vi "Send  Sensor Calibration.vi"(6 "Initialize/Close?":bool, 8 "Error In (No Error)":errorcluster, 9 "Sensor On/Off":bool, 10 "Sensor Address In":string="0", 11 "RS232 Port In":refnum<visa-resource-name>="COM11") -> (0 "Error Out":errorcluster, 1 "Sensor On/Off Response":bool, 2 "Address Out":string, 3 "RS232 Port Out":refnum<visa-resource-name>)   [LabVIEW 2016]
doc: "Sends an SDI-12 Send Identification Command, and returns the various attributes from the sensor's response.\n\nThe total size by the sensor must be 22-35 in size (inclusive), or this VI will return an error."
uses:
  SDI-12/SDI-12.lvlib
panel:
  out "Numeric":i32
  out "read buffer":string
  out "length":i32
  out "output 1":i16
  out "Command":string
  # "(c) 2008 National Instruments.  ALL RIGHTS RESERVED."
  # "The following are required,\nor are optional, for the sensors\nto respond with:"
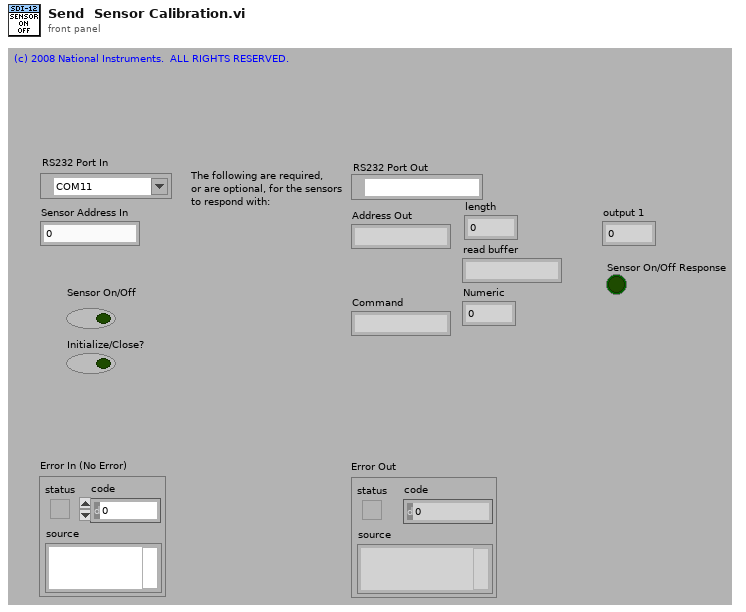
[diagram p1: front panel]
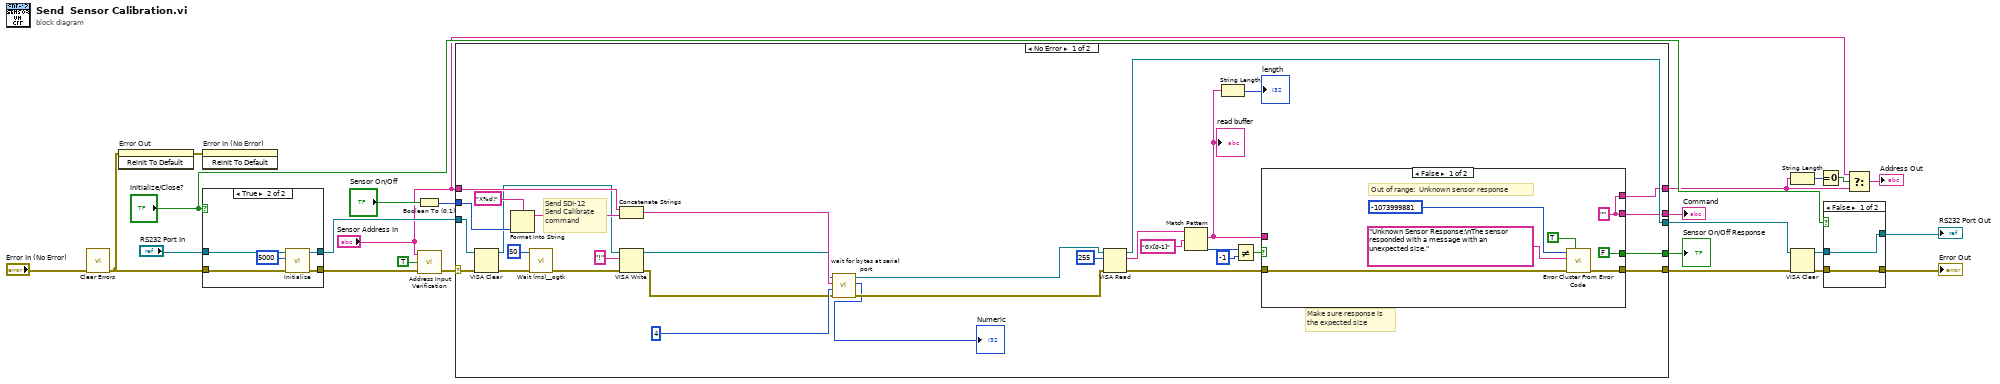
[diagram p0: block diagram]
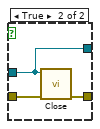
[diagram p2: hidden frame]
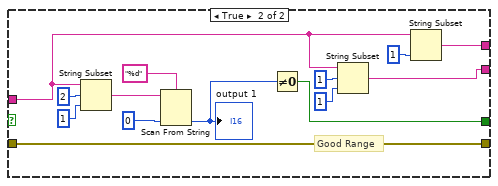
[diagram p4: hidden frame]
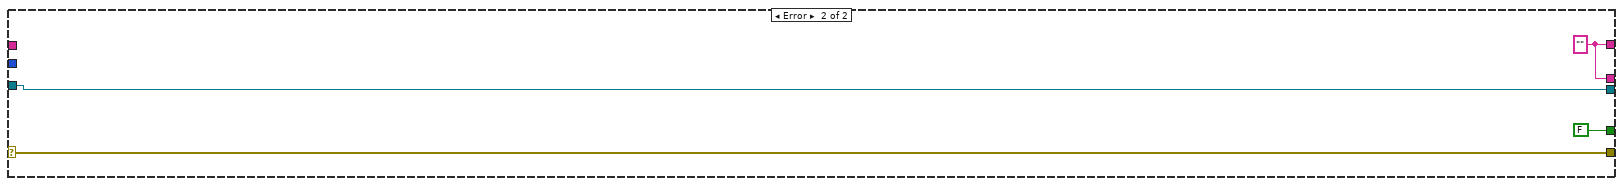
[diagram p5: hidden frame]
diagram:
  n1 = call <vilib>:"Clear Errors.vi"("error in (no error)"="Error In (No Error)") -> ("error out"=w5:errorcluster)  [unwired: 5 in, 1 out]
  n2 = invoke on="Error Out" class="Clust (strict)" method="Reinit To Default"(error in=w5) -> (error out=w4:errorcluster)  [unwired: 2 in, 2 out]
  n3 = invoke on="Error In (No Error)" class="Clust (strict)" method="Reinit To Default"(error in=w4) -> ()  [unwired: 2 in, 3 out]
  n4 = case shown="True" "Initialize/Close?" {
    tunnel: w5 -> [w26 w31]
    tunnel: [w26 w30] -> w16
    tunnel: "RS232 Port In" -> [w25 w29]
    tunnel: [w25 w28] -> w15
    frame False {
    }
    frame True {
      n5 = call "Initialize.vi"("Error In (No Error)"=w31, "General Settings:Timeout Value"=u32 5000, "RS232 Port In"=w29) -> ("Error Out"=w30:errorcluster, "RS232 Port Out"=w28:refnum<visa-resource-name>)  [unwired: 7 in]
    }
  }
  n6 = Boolean To (0,1)(Boolean="Sensor On/Off") -> (0, 1=w20:i16)
  n7 = call "Address Input Verification.vi"("Error In (No Error)"=w16, "Error if Bad? (True)"=TRUE ("error if bad? (True)"), "Sensor Address In (a)"="Sensor Address In") -> ("Error Out"=w24:errorcluster)  [unwired: 1 in, 1 out]
  n8 = case shown="No Error" w24 {
    selector: w24 -> [w50 w88]
    tunnel: [w58 w88] -> w2
    tunnel: "Sensor Address In" -> [w62 _]
    tunnel: w15 -> [w51 w87]
    tunnel: [w61 w87] -> w13
    tunnel: [w57 w86] -> w22
    tunnel: [w56 w86] -> w8
    tunnel: w20 -> [w55 _]
    tunnel: [w52 FALSE] -> w19
    frame No Error {
      # "Make sure response is\nthe expected size"
      # "Send SDI-12 \nSend Calibrate \ncommand"
      n9 = VISA Clear(VISA resource name=w51, error in (no error)=w50) -> (VISA resource name out=w41:refnum<visa-resource-name>, error out=w45:errorcluster)
      n10 = Format Into String(format string="X%d!", w55) -> (resulting string=w53:string)  [unwired: 2 in, 1 out]
      n11 = call "Wait (ms)__ogtk.vi"("error in (no error)"=w45, "milliseconds to wait"=u32 50) -> ("error out"=w42:errorcluster)  [unwired: 8 in, 1 out]
      n12 = Concatenate Strings(w62, w53) -> (w49:string)
      n13 = VISA Write(VISA resource name=w41, write buffer="!", error in (no error)=w42) -> (VISA resource name out=w33:refnum<visa-resource-name>, error out=w40:errorcluster)  [unwired: 1 out]
      n14 = call "wait for bytes at serial port.vi"("error in (no error)"=w40, "lower limit"=4, "String"=w49, "VISA Refnum in"=w33) -> ("error out"=w47:errorcluster, "loop"=→"Numeric":i32, "VISA Refnum out"=w48:refnum<visa-resource-name>)  [unwired: 4 in, 1 out]
      n15 = VISA Read(VISA resource name=w48, byte count=u32 255, error in (no error)=w47) -> (VISA resource name out=w61:refnum<visa-resource-name>, read buffer=w59:string, error out=w60:errorcluster)  [unwired: 1 out]
      n16 = Match Pattern(string=w59, regular expression="0X[0-1]") -> (match substring=w38:string, offset past match=w36:i32)  [unwired: 1 in, 2 out]
      "read buffer" <- w38
      n17 = String Length(string=w38) -> (length=→"length":i32)
      n18 = Not Equal?(x=w36, y=-1) -> (x != y?=w34:bool)
      n19 = case shown="False" w34 {
        tunnel: w60 -> [w66 w78]
        tunnel: [w67 w78] -> w58
        tunnel: w38 -> [_ w81]
        tunnel: [w65 w76] -> w57
        tunnel: [w65 w75] -> w56
        tunnel: [FALSE w71] -> w52
        frame False {
          w65 = "" ("read buffer")
          # "Out of range:  Unknown sensor response"
          n20 = call <vilib>:"Error Cluster From Error Code.vi"("show call chain? (False)"=TRUE, "error in (no error)"=w66, "error message (\"\")"="Unknown Sensor Response:\nThe sensor responded with a message with an unexpected size." ("error message (\"\")"), "error code (0)"=-1073999881) -> ("error out"=w67:errorcluster)  [unwired: 5 in]
        }
        frame True {
          # "Good Range"
          n21 = String Subset(string=w81, offset (0)=2, length (rest)=1 ("length (rest)")) -> (substring=w77:string)
          n22 = Scan From String(format string="%d", input string=w77, default 1=i16 0 ("default value 1")) -> (output 1=w72:i16)  [unwired: 2 in, 3 out]
          "output 1" <- w72
          n23 = Not Equal To 0?(x=w72) -> (x != 0?=w71:bool)
          n24 = String Subset(string=w81, offset (0)=1, length (rest)=1 ("length (rest)")) -> (substring=w76:string)
          n25 = String Subset(string=w81, length (rest)=1 ("length (rest)")) -> (substring=w75:string)  [unwired: 1 in]
        }
      }
    }
    frame Error {
      w86 = "" ("read buffer")
    }
  }
  "Command" <- w22
  "Sensor On/Off Response" <- w19
  n26 = String Length(string=w8) -> (length=w10:i32)
  n27 = VISA Clear(VISA resource name=w13, error in (no error)=w2) -> (VISA resource name out=w3:refnum<visa-resource-name>, error out=w1:errorcluster)
  n28 = Equal To 0?(x=w10) -> (x = 0?=w9:bool)
  n29 = case shown="False" "Initialize/Close?" {
    tunnel: w1 -> [w90 w93]
    tunnel: [w90 w92] -> w14
    tunnel: w3 -> [w89 w91]
    tunnel: [w89 w91] -> w12
    frame False {
    }
    frame True {
      n30 = call "Close.vi"("Error In (No Error)"=w93, "RS232 Port In"=w91) -> ("Error Out"=w92:errorcluster)  [unwired: 9 in]
    }
  }
  "Error Out" <- w14
  "RS232 Port Out" <- w12
  n31 = Select(t="Sensor Address In", s=w9, f=w8) -> (s? t:f=→"Address Out":string)
